vi "Send Telnet Message.vi"(8 "error in":errorcluster, 10 "Message In":string, 11 "Telnet V2 in":refnum<class "Telnet V2.lvclass">) -> (0 "error out":errorcluster)   [LabVIEW 2018, in "Telnet V2.lvlib" / "Telnet V2.lvclass"]
uses:
  Telnet V2.lvclass
  Telnet V2.lvclass/Telnet V2.ctl
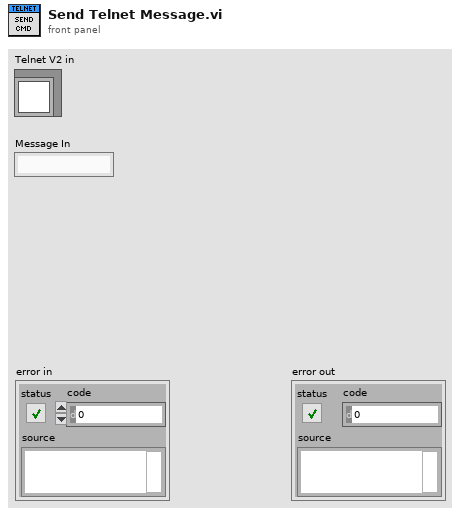
[diagram p1: front panel]
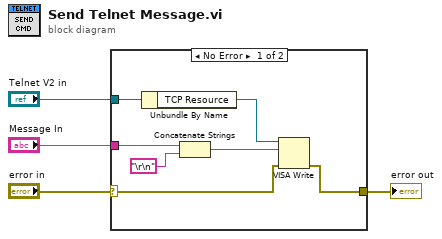
[diagram p0: block diagram]
diagram:
  n1 = case shown="No Error" "error in" {
    selector: "error in" -> [w6 w12]
    tunnel: "Telnet V2 in" -> [w8 _]
    tunnel: "Message In" -> [w10 _]
    tunnel: [w5 w12] -> w1
    frame No Error {
      n2 = Unbundle By Name(w8) -> ("TCP Resource"=w7:refnum<visa-resource-name>)
      n3 = Concatenate Strings(w10, "\r\n") -> (w9:string)
      n4 = VISA Write(VISA resource name=w7, write buffer=w9, error in (no error)=w6) -> (error out=w5:errorcluster)  [unwired: 2 out]
    }
    frame Error {
    }
  }
  "error out" <- w1
